vi "Inst UI.Krohn-Hite-7008.TestLauncher.vi"() -> ()   [LabVIEW 2019, in "Inst UI.Krohn-Hite-7008.lvclass"]
doc: "JKI State Machine Objects (SMO) 1.0.0.5\nJKI - JKI\nCopyright (c) 2016, JKI"
uses:
  Inst UI.Krohn-Hite-7008.lvclass
  C:/Program Files (x86)/National Instruments/LabVIEW 2019/vi.lib/JKI/JKI SMO/SMO/SMO.lvclass
  C:/Program Files (x86)/National Instruments/LabVIEW 2019/vi.lib/JKI/JKI SMO/SMO.UI/SMO.UI.lvclass
  <vilib>/JKI/JKI SMO/SMO/SMO.lvclass/SMO.ctl
  <vilib>/JKI/JKI SMO/SMO.UI/SMO.UI.lvclass/SMO.UI.ctl
  <vilib>/JKI/JKI SMO/SMO/Typedefs/SMOState --Enum.ctl
  <vilib>/JKI/JKI SMO/SMO/Private/ReftoDVR--SMO.vi
  <vilib>/JKI/JKI SMO/SMO.UI/SMO.UI.ReftoDVR.vi
  <vilib>/JKI/JKI SMO/SMO/SMO.lvclass
  <vilib>/JKI/JKI SMO/SMO.UI/SMO.UI.lvclass
panel:
  out "error out":errorcluster
  in  "Stop":bool
  # "SMO UI Test Launcher"
  # "For instructions on how to use the JKI State Machine Objects, examples and video tutorials, visit:\nhttp://jki.net/state-machine-objects/\n\nJKI State Machine Objects™\nhttp://jki.net/state-machine-objects/\nCopyright (C) 2005-2015, JKI <info@jki.net>\nALL RIGHTS RESERVED"
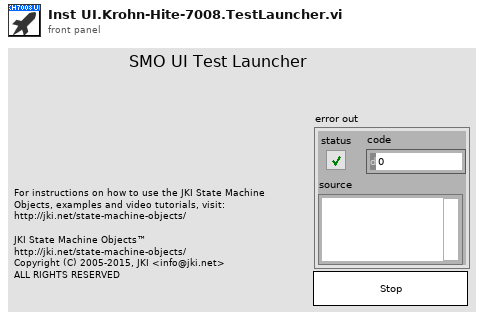
[diagram p1: front panel]
types:
  T1 = typedef "SMO.lvclass/Public Events.ctl" = cluster{"Error":refnum<user-event>, "State":refnum<user-event>, "Reserve State":refnum<user-event>}
  T2 = typedef "SMO.UI.lvclass/PublicEvents--Cluster.ctl" = cluster{"UI Hidden":refnum<user-event>, "UI State":refnum<user-event>}
  T3 = typedef "SMO.lvclass/SMOState --Enum.ctl" = enum16{"unknown", "Created", "Started", "Stopped"}
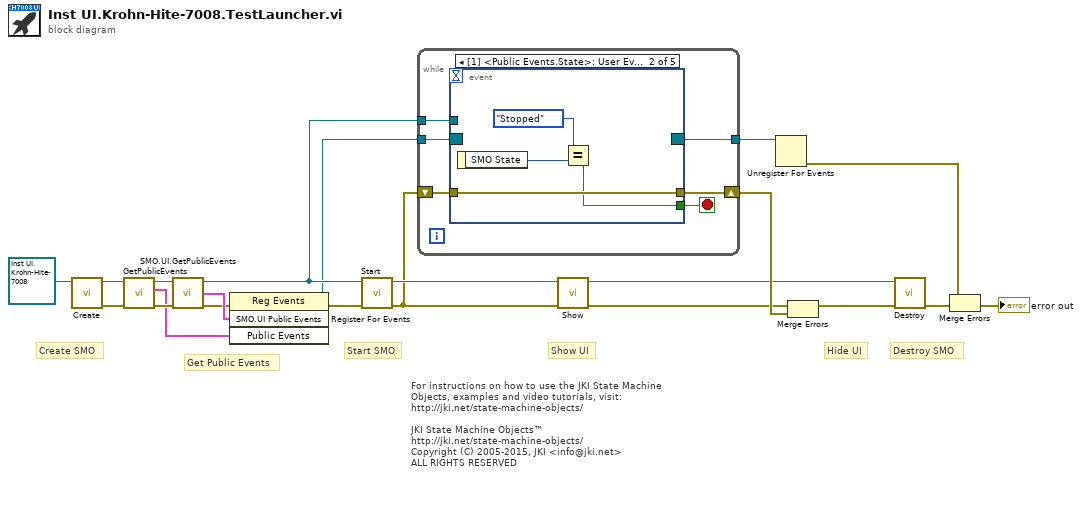
[diagram p0: block diagram]
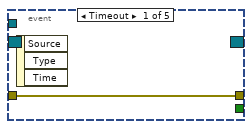
[diagram p2: hidden frame]
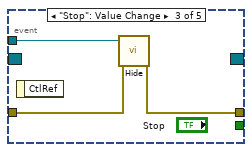
[diagram p3: hidden frame]
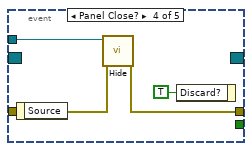
[diagram p4: hidden frame]
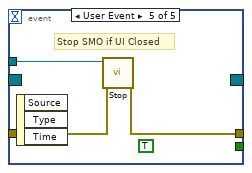
[diagram p5: hidden frame]
diagram:
  # "Hide UI"
  # "Show UI"
  # "For instructions on how to use the JKI State Machine Objects, examples and video tutorials, visit:\nhttp://jki.net/state-machine-objects/\n\nJKI State Machine Objects™\nhttp://jki.net/state-machine-objects/\nCopyright (C) 2005-2015, JKI <info@jki.net>\nALL RIGHTS RESERVED"
  # "Get Public Events"
  # "Start SMO"
  # "Destroy SMO"
  # "Create SMO"
  n1 = call <vilib>:"Create.vi"("SMO"=refnum<class "Inst UI.Krohn-Hite-7008.lvclass"> refnum ("SMO.Template.lvclass")) -> ("error out"=w5:errorcluster, "SMO out"=w4:refnum<class "Inst UI.Krohn-Hite-7008.lvclass">)  [unwired: 8 in, 1 out]
  n2 = call <vilib>:"GetPublicEvents.vi"("error in (no error)"=w5, "SMO"=w4) -> ("error out"=w2:errorcluster, "Public Events"=w1:T1, "SMO out"=w3:refnum<class "Inst UI.Krohn-Hite-7008.lvclass">)  [unwired: 7 in]
  n3 = call <vilib>:"SMO.UI.GetPublicEvents.vi"("error in (no error)"=w2, "SMO.UI"=w3) -> ("error out"=w8:errorcluster, "SMO.UI Public Events"=w9:T2, "SMO.UI out"=w10:refnum<class "Inst UI.Krohn-Hite-7008.lvclass">)  [unwired: 7 in]
  n4 = register-events(error in=w8, w9, w1) -> (reference out=w6:refnum<event-registration>, error out=w7:errorcluster)  [unwired: 1 in]
  n5 = call <vilib>:"Start.vi"("error in (no error)"=w7, "SMO"=w10) -> ("error out"=w14:errorcluster, "SMO out"=w15:refnum<class "Inst UI.Krohn-Hite-7008.lvclass">)  [unwired: 8 in]
  n6 = while {
    shift-right: [w26] -> w20
    shift-left: w14 -> [w25]
    tunnel: w6 -> [w24]
    tunnel: [w23] -> w21
    tunnel: w10 -> [w22]
    stop <- w27 stop-if-true
    n7 = event shown="[1] <Public Events.State>: User Event" {
      selector: w24 -> [_ _ _ _ _]
      dyn-events: [_ _ _ _ _] -> w23
      timeout: _ -> [_ _ _ _ _]
      tunnel: [_ w29 _ _ _] -> w27
      tunnel: w22 -> [_ _ w35 w38 w42]
      tunnel: [w28 w32 w33 w36 w41] -> w26
      tunnel: w25 -> [w28 w32 w34 w37 w40]
      event Timeout {
        n8 = event-data() -> ()  [unwired: 1 in, 3 out]
      }
      event User Event {
        n9 = event-data() -> ("SMO State"=w31:T3)  [unwired: 1 in]
        n10 = Equal?(x=SMOState_--Enum."Stopped", y=w31) -> (x = y?=w29:bool)
      }
      event "Stop": Value Change {
        n11 = event-data() -> ()  [unwired: 1 in, 1 out]
        n12 = call <vilib>:"Hide.vi"("error in (no error)"=w34, "SMO.UI"=w35) -> ("error out"=w33:errorcluster)  [unwired: 8 in, 1 out]
      }
      event Panel Close? {
        n13 = event-data() -> ()  [unwired: 1 in, 1 out]
        n14 = call <vilib>:"Hide.vi"("error in (no error)"=w37, "SMO.UI"=w38) -> ("error out"=w36:errorcluster)  [unwired: 8 in, 1 out]
        n15 = event-data("Discard?"=TRUE ("OK")) -> ()  [unwired: 1 in, 1 out]
      }
      event User Event {
        (unwired) TRUE ("OK")
        # "Stop SMO if UI Closed"
        n16 = event-data() -> ()  [unwired: 1 in, 3 out]
        n17 = call <vilib>:"Stop.vi"("error in (no error)"=w40, "SMO"=w42) -> ("error out"=w41:errorcluster)  [unwired: 8 in, 1 out]
      }
    }
  }
  n18 = call <vilib>:"Show.vi"("error in (no error)"=w14, "SMO.UI"=w15) -> ("error out"=w13:errorcluster, "SMO.UI out"=w12:refnum<class "Inst UI.Krohn-Hite-7008.lvclass">)  [unwired: 8 in]
  n19 = Unregister For Events(event registration refnum=w21) -> (error out=w19:errorcluster)  [unwired: 1 in]
  n20 = Merge Errors(w13, w20) -> (w11:errorcluster)
  n21 = call <vilib>:"Destroy.vi"("error in (no error)"=w11, "SMO"=w12) -> ("error out"=w17:errorcluster)  [unwired: 9 in]
  n22 = Merge Errors(w19, w17) -> (→"error out":errorcluster)
